vi "niScope Add Waveform Processing.vi"(0 "instrument handle":refnum<k15>, 5 "channels":string="0", 9 "array measurement":T1=4000 items=["None"=4000, "Last Acq. Histogram"=4001, "Multi Acq. Voltage Histogram"=4004, "Multi Acq. Time Histogram"=4005, "Multi Acq. Average"=4016, "Polynomial Interpolation"=4011, "Array Integral"=4006, "Derivative"=4007, "Inverse"=4008, "Multiply Channels"=4012, "Add Channels"=4013, "Subtract Channels"=4014, "Divide Channels"=4015, "Array Offset"=4025, "Array Gain"=4026, "Hanning Window"=4009, "Flat Top Window"=4010, "Hamming Window"=4020, "Triangle Window"=4023, "Blackman Window"=4024, "FIR Windowed Filter"=4021, "Bessel IIR Filter"=4022, "Butterworth IIR Filter"=4017, "Chebyshev IIR Filter"=4018, "FFT Phase Spectrum"=4002, "FFT Amp. Spectrum (Volts RMS)"=4003, "FFT Amp. Spectrum (dB)"=4019], 11 "error in":errorcluster) -> (4 "instrument handle out":refnum<k15>, 15 "error out":errorcluster)   [LabVIEW 2013]
doc: "Adds one measurement to the list of processing steps that are completed before the measurement. The processing is added on a per channel basis, and the processing measurements are completed in the same order they are registered. All waveform measurements (for example, adding channels or applying a Bessel filter) are cached at the time of registering the processing, and this set of measurements is used during the processing step. The processing measurements are streamed, so the result of the first processing step is used as the input for the next step. The processing happens before any other measurements."
uses:
  <instrlib>/niScope/Controls/niScope array measurement.ctl
  niScope_32.dll
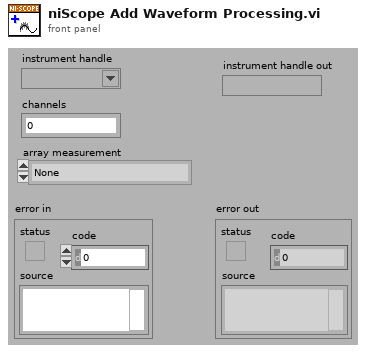
[diagram p1: front panel]
types:
  T1 = typedef "niScope array measurement.ctl" = i32
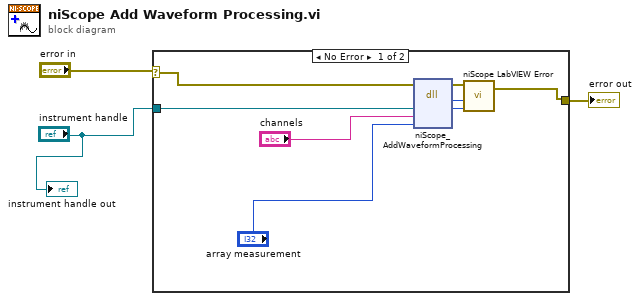
[diagram p0: block diagram]
diagram:
  n1 = case shown="No Error" "error in" {
    selector: "error in" -> [w4 w11]
    tunnel: [w5 w11] -> w2
    tunnel: "instrument handle" -> [w10 _]
    frame No Error {
      n2 = dll-call lib="niScope_*.*" fn="niScope_AddWaveformProcessing"("instrument handle"=w10, "channel"="channels", "measFunction"="array measurement") -> ("status"=w6:i32, "instrument handle"=w7:u32)  [unwired: 5 in, 2 out]
      n3 = call <instrlib>:"niScope LabVIEW Error.vi"("instrument handle"=w7, "niScope error code (0)"=w6, "error in (no error)"=w4) -> ("error out"=w5:errorcluster)  [unwired: 2 in]
    }
    frame Error {
    }
  }
  "error out" <- w2
  "instrument handle out" <- "instrument handle"
